vi "Write Pressure.vi"(8 "error in (no error)":errorcluster, 10 "Pressure":dbl, 11 "Open Path Data in":refnum<class "Open Path Data.lvclass">) -> (0 "error out":errorcluster, 3 "Open Path Data out":refnum<class "Open Path Data.lvclass">)   [LabVIEW 2015, in "Open Path Data.lvclass"]
uses:
  Open Path Data.lvclass
  Open Path Data.lvclass/Open Path Data.ctl
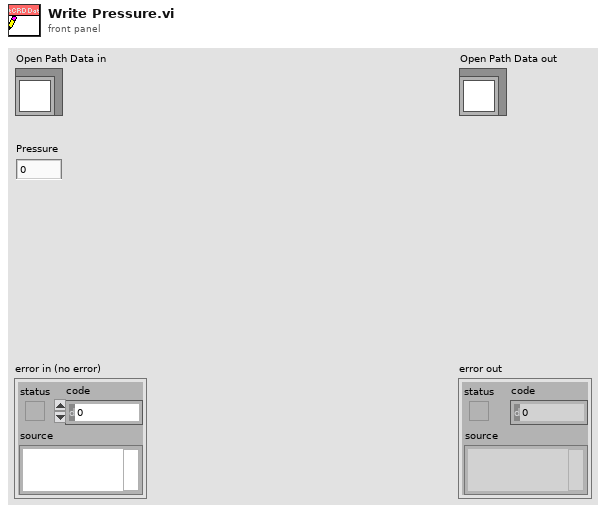
[diagram p1: front panel]
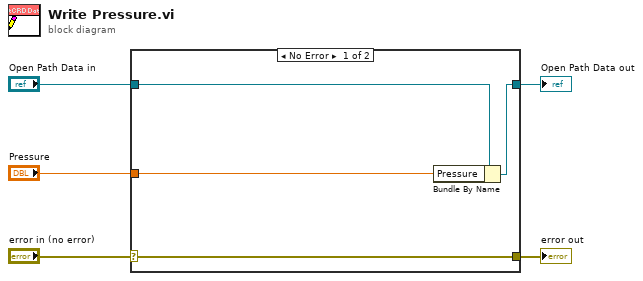
[diagram p0: block diagram]
diagram:
  n1 = case shown="No Error" "error in (no error)" {
    selector: "error in (no error)" -> [w9 w10]
    tunnel: [w9 w10] -> w4
    tunnel: [w7 w11] -> w2
    tunnel: "Open Path Data in" -> [w8 w11]
    tunnel: "Pressure" -> [w6 _]
    frame No Error {
      n2 = Bundle By Name(cluster=w8, "Pressure"=w6) -> (w7:refnum<class "Open Path Data.lvclass">)
    }
    frame Error {
    }
  }
  "error out" <- w4
  "Open Path Data out" <- w2
